vi "Reinterpret I32 as U32.vi"(7 "Input":i32) -> (8 "Output":u32)   [LabVIEW 2012]
uses:
  <vilib>/rvi/FXPMathLib/FxpInterpret/XNode/nifxpmath_Interpret.xnode
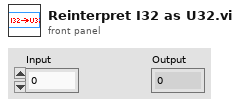
[diagram p1: front panel]
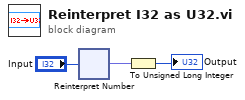
[diagram p0: block diagram]
diagram:
  n1 = xnode "Reinterpret Number"("x"="Input") -> ("y"=w3:fxp<+/-,32,32>)
  n2 = To Unsigned Long Integer(number=w3) -> (unsigned 32bit integer=→"Output":u32)
